vi "_Update Mass Range.vi"(4 "error in":errorcluster, 5 "Mass Range":T1 {"Resolution Type" items=["High/High", "Medium/Medium", "Low/Low", "High/Medium", "High/Low", "Medium/High", "Medium/Low", "Low/High", "Low/Medium"]}, 6 "Offset":u16) -> (0 "error out":errorcluster, 2 "Next Offset":u16)   [LabVIEW 2012]
uses:
  Type/_RT Mass Range.ctl
  Type/_RT Res Type.ctl
  Type/_RT Active Ch.ctl
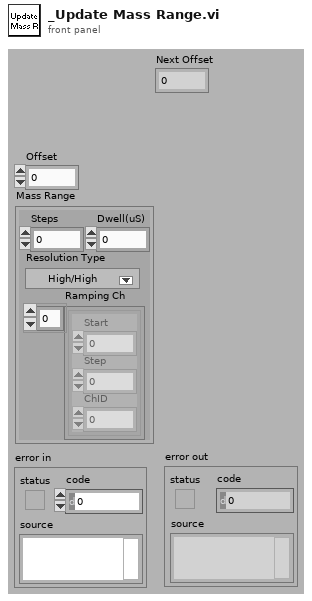
[diagram p1: front panel]
types:
  T1 = typedef "_RT Mass Range.ctl" = cluster{"Steps":i32, "Dwell(uS)":i32, "Resolution Type":T2, "Ramping Ch":T3[]}
  T2 = typedef "_RT Res Type.ctl" = u16
  T3 = typedef "_RT Active Ch.ctl" = cluster{"Start":i32, "Step":i32, "ChID":i32}
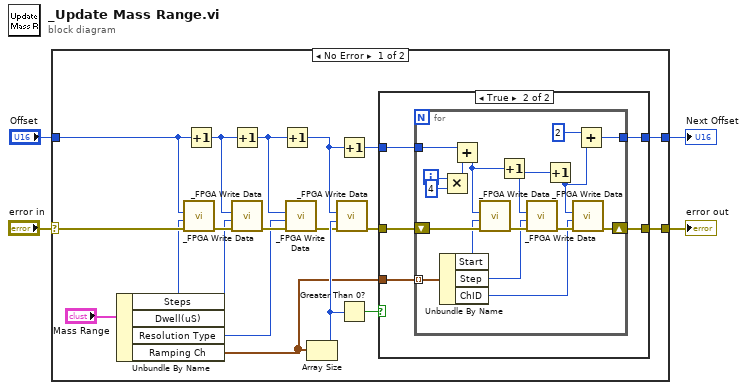
[diagram p0: block diagram]
diagram:
  n1 = case shown="No Error" "error in" {
    selector: "error in" -> [w21 w49]
    tunnel: [w13 w49] -> w3
    tunnel: "Offset" -> [w17 w48]
    tunnel: [w11 w48] -> w1
    frame No Error {
      n2 = Unbundle By Name("Mass Range") -> ("Steps"=w20:i32, "Dwell(uS)"=w18:i32, "Resolution Type"=w7:T2, "Ramping Ch"=w10:T3[])
      n3 = call "_FPGA Write Data.vi"("error in"=w21, "Data"=w20, "Address"=w17) -> ("error out"=w22:errorcluster)  [unwired: 3 in, 2 out]
      n4 = Increment(x=w17) -> (x+1=w19:u16)
      n5 = Increment(x=w19) -> (x+1=w8:u16)
      n6 = call "_FPGA Write Data.vi"("error in"=w22, "Data"=w18, "Address"=w19) -> ("error out"=w9:errorcluster)  [unwired: 3 in, 2 out]
      n7 = Increment(x=w8) -> (x+1=w5:u16)
      n8 = call "_FPGA Write Data.vi"("error in"=w9, "Data"=w7, "Address"=w8) -> ("error out"=w6:errorcluster)  [unwired: 3 in, 2 out]
      n9 = Array Size(array=w10) -> (size(s)=w16:i32)
      n10 = call "_FPGA Write Data.vi"("error in"=w6, "Data"=w16, "Address"=w5) -> ("error out"=w14:errorcluster)  [unwired: 3 in, 2 out]
      n11 = Increment(x=w5) -> (x+1=w12:u16)
      n12 = Greater Than 0?(x=w16) -> (x > 0?=w15:bool)
      n13 = case shown="True" w15 {
        tunnel: [w25 w27] -> w13
        tunnel: w14 -> [w25 w29]
        tunnel: w12 -> [w24 w28]
        tunnel: [w24 w26] -> w11
        tunnel: w10 -> [_ w30]
        frame False {
        }
        frame True {
          n14 = for {
            tunnel: w30 -> [w43] mode=indexing
            shift-right: [w34] -> w27
            shift-left: w29 -> [w42]
            tunnel: w28 -> [w44]
            tunnel: [w32] -> w26
            i -> [w47]
            n15 = Unbundle By Name(w43) -> ("Start"=w41:i32, "Step"=w39:i32, "ChID"=w35:i32)
            n16 = Multiply(x=w47, y=4) -> (x*y=w45:i32)
            n17 = Add(x=w44, y=w45) -> (x+y=w38:i32)
            n18 = call "_FPGA Write Data.vi"("error in"=w42, "Data"=w41, "Address"=w38) -> ("error out"=w40:errorcluster)  [unwired: 3 in, 2 out]
            n19 = Increment(x=w38) -> (x+1=w36:i32)
            n20 = call "_FPGA Write Data.vi"("error in"=w40, "Data"=w39, "Address"=w36) -> ("error out"=w37:errorcluster)  [unwired: 3 in, 2 out]
            n21 = Increment(x=w36) -> (x+1=w33:i32)
            n22 = call "_FPGA Write Data.vi"("error in"=w37, "Data"=w35, "Address"=w33) -> ("error out"=w34:errorcluster)  [unwired: 3 in, 2 out]
            n23 = Add(x=2, y=w33) -> (x+y=w32:i32)
          }
        }
      }
    }
    frame Error {
    }
  }
  "error out" <- w3
  "Next Offset" <- w1
